vi "SetLiftHome.vi"(8 "error in (no error)":errorcluster) -> (0 "error out":errorcluster)   [LabVIEW 2014]
uses:
  Gantry/GantryGlobals.vi
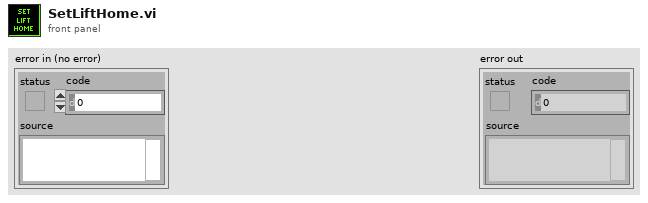
[diagram p1: front panel]
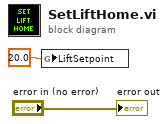
[diagram p0: block diagram]
diagram:
  n1 = global write "GantryGlobals.vi" "LiftSetpoint"(20.0 ("LiftSetpoint")) -> ()
  "error out" <- "error in (no error)"
